vi "NMIdleLoop.vi"(1 "ULx task in":refnum<k24>, 2 "Tab Control":enum32{"ULx", "DAQmx"}(tab), 5 "error in":errorcluster, 6 "Start":bool, 8 "ExStop":bool, 10 "ExClear":bool) -> (7 "Task Start":bool, 9 "Task Stop":bool, 11 "Task Clear":bool, 15 "ULx task out":refnum<k24>, 17 "Task":i32 format="%x", 18 "Function":i32, 19 "error out":errorcluster)   [LabVIEW 2010]
uses:
  C:/Program Files/National Instruments/LabVIEW 2010/vi.lib/ULx/ULx_LV.dll
  Program Files/National Instruments/LabVIEW 2010/vi.lib/ULx/ULx_LV.dll
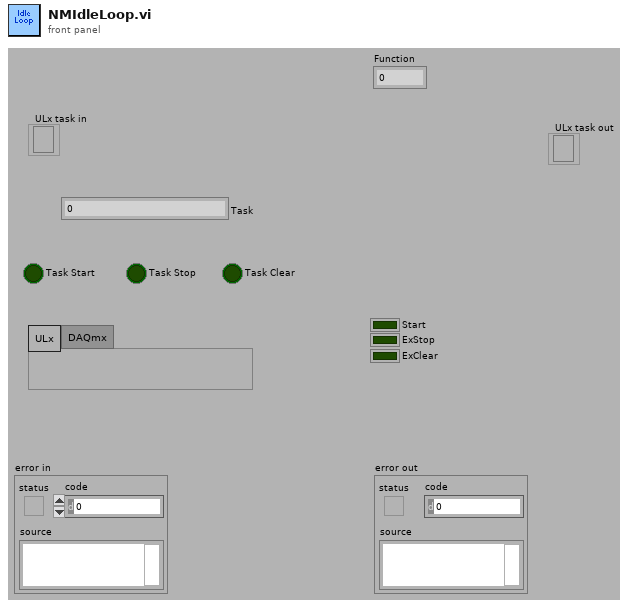
[diagram p1: front panel]
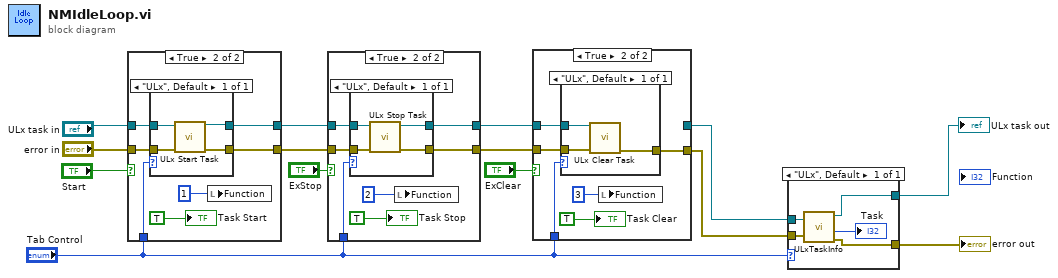
[diagram p0: block diagram]
diagram:
  n1 = case shown="True" "Start" {
    tunnel: [w16 w23] -> w4
    tunnel: "ULx task in" -> [w16 w22]
    tunnel: "error in" -> [w15 w21]
    tunnel: [w15 w20] -> w5
    tunnel: "Tab Control" -> [_ w19]
    frame False {
    }
    frame True {
      n2 = case shown="\"ULx\", Default" w19 {
        tunnel: [w27] -> w23
        tunnel: w22 -> [w26]
        tunnel: w21 -> [w25]
        tunnel: [w24] -> w20
        frame "ULx", Default {
          n3 = call <vilib>:"ULx Start Task.vi"("task in"=w26, "error in"=w25) -> ("task out"=w27:refnum<k24>, "error out"=w24:errorcluster)  [unwired: 12 in]
        }
      }
      n4 = local write "Function"(1) -> ()
      "Task Start" <- TRUE
    }
  }
  n5 = case shown="True" "ExStop" {
    tunnel: [w29 w36] -> w9
    tunnel: w4 -> [w29 w35]
    tunnel: w5 -> [w28 w34]
    tunnel: [w28 w33] -> w8
    tunnel: "Tab Control" -> [_ w32]
    frame False {
    }
    frame True {
      n6 = case shown="\"ULx\", Default" w32 {
        tunnel: [w40] -> w36
        tunnel: w35 -> [w39]
        tunnel: w34 -> [w38]
        tunnel: [w37] -> w33
        frame "ULx", Default {
          n7 = call <vilib>:"ULx Stop Task.vi"("error in"=w38, "task in"=w39) -> ("error out"=w37:errorcluster, "task out"=w40:refnum<k24>)  [unwired: 8 in]
        }
      }
      n8 = local write "Function"(2) -> ()
      "Task Stop" <- TRUE
    }
  }
  n9 = case shown="True" "ExClear" {
    tunnel: w9 -> [w41 w48]
    tunnel: w8 -> [w42 w47]
    tunnel: [w42 w46] -> w1
    tunnel: "Tab Control" -> [_ w45]
    tunnel: [w41 _] -> w11
    frame False {
    }
    frame True {
      n10 = case shown="\"ULx\", Default" w45 {
        tunnel: w48 -> [w49]
        tunnel: w47 -> [w51]
        tunnel: [w50] -> w46
        frame "ULx", Default {
          n11 = call <vilib>:"ULx Clear Task.vi"("task in"=w49, "error in"=w51) -> ("error out"=w50:errorcluster)  [unwired: 13 in]
        }
      }
      n12 = local write "Function"(3) -> ()
      "Task Clear" <- TRUE
    }
  }
  n13 = case shown="\"ULx\", Default" "Tab Control" {
    tunnel: w11 -> [w56]
    tunnel: w1 -> [w54]
    tunnel: [w53] -> w3
    tunnel: [w52] -> w2
    frame "ULx", Default {
      n14 = call "ULxTaskInfo.vi"("task in"=w56, "error in (no error)"=w54) -> ("task in 2"=w52:refnum<k24>, "Task"=→"Task":i32, "error out"=w53:errorcluster)  [unwired: 2 out]
    }
  }
  "ULx task out" <- w2
  "error out" <- w3
